vi "Get Front Panel Info.vi"(8 "error in":errorcluster, 11 "VI in":refnum<vi>) -> (0 "error out":errorcluster, 2 "label array out":string[](array[string]), 3 "Controls[]":refnum<vi>[](array[refnum]), 4 "width":i16, 5 "panel ref out":refnum<vi>, 6 "height":i16)   [LabVIEW 2018]
uses:
  <vilib>/Utility/miscctls.llb/LVPointTypeDef.ctl
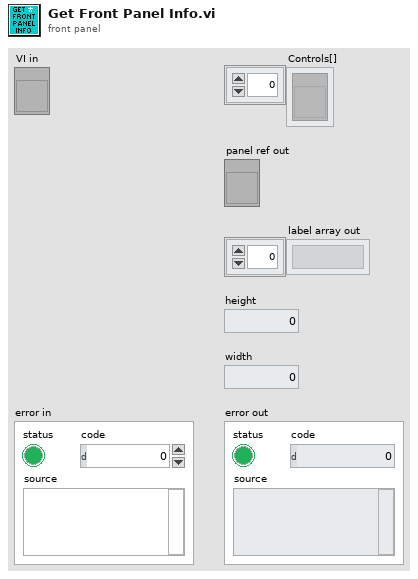
[diagram p1: front panel]
types:
  T1 = typedef "LVPointTypeDef.ctl" = cluster{"Horizontal":i16, "Vertical":i16}
  T2 = typedef "LVRectTypeDef.ctl" = cluster{"Left":i16, "Top":i16, "Right":i16, "Bottom":i16}
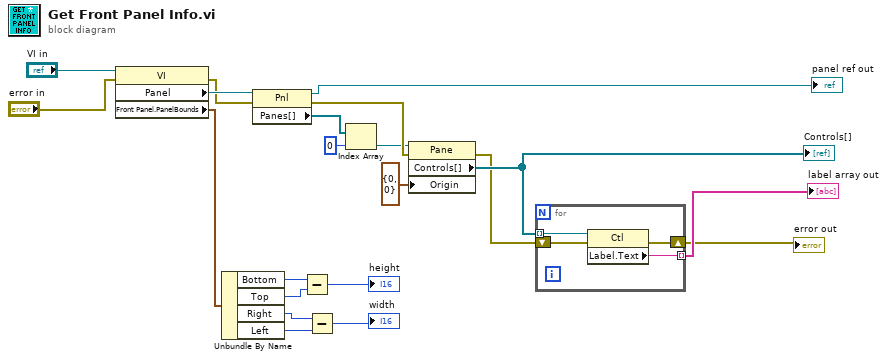
[diagram p0: block diagram]
diagram:
  n1 = property class="VI"(reference="VI in", error in="error in") -> (error out=w10:errorcluster, "Panel"=w18:refnum<vi>, "Front Panel.PanelBounds"=w13:T2)  [unwired: 1 out]
  n2 = Unbundle By Name(w13) -> ("Bottom"=w16:i16, "Top"=w17:i16, "Right"=w20:i16, "Left"=w21:i16)
  n3 = property class="Pnl"(reference=w18, error in=w10) -> (reference out=→"panel ref out":refnum<vi>, error out=w11:errorcluster, "Panes[]"=w9:refnum<vi>[])
  n4 = Subtract(x=w16, y=w17) -> (x-y=→"height":i16)
  n5 = Subtract(x=w20, y=w21) -> (x-y=→"width":i16)
  n6 = Index Array(array=w9, index=0) -> (element=w8:refnum<vi>)
  n7 = property class="Pane"(reference=w8, error in=w11, "Origin"=T1 {"Horizontal"=0, "Vertical"=0}) -> (error out=w12:errorcluster, "Controls[]"=w14:refnum<vi>[])  [unwired: 1 out]
  "Controls[]" <- w14
  n8 = for {
    tunnel: w14 -> [w23] mode=indexing
    shift-right: [w24] -> w4
    shift-left: w12 -> [w25]
    tunnel: [w22] -> w15 mode=indexing
    n9 = property class="Ctl"(reference=w23, error in=w25) -> (error out=w24:errorcluster, "Label.Text"=w22:string)  [unwired: 1 out]
  }
  "error out" <- w4
  "label array out" <- w15
